vi "is a.vi"(8 "error in (no error)":errorcluster, 11 "TempController in":refnum<class "TempController.lvclass">) -> (0 "error out":errorcluster, 2 "is a":string, 3 "TempController out":refnum<class "TempController.lvclass">)   [LabVIEW 2016, in "Hardware.lvlib" / "TempController.lvclass"]
uses:
  <userlib>/Common Components/Hardware/TempController/TempController.lvclass
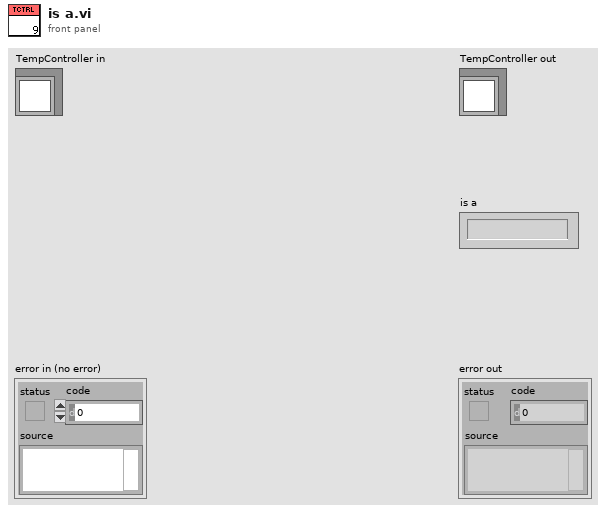
[diagram p1: front panel]
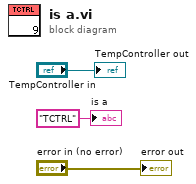
[diagram p0: block diagram]
diagram:
  "error out" <- "error in (no error)"
  "TempController out" <- "TempController in"
  "is a" <- "TCTRL" ("is a")
